vi "moveabs2.vi"(2 "SetPosition":sgl format="%.2f", 3 "EXP300 Axis":i8=1, 4 "THz Image\nESP Address":string="1:1") -> (0 "Current Position":dbl)   [LabVIEW 2010]
panel:
  out "Time to wait (s)":i16
  # "Stage Moving"
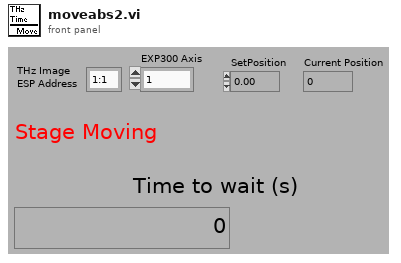
[diagram p1: front panel]
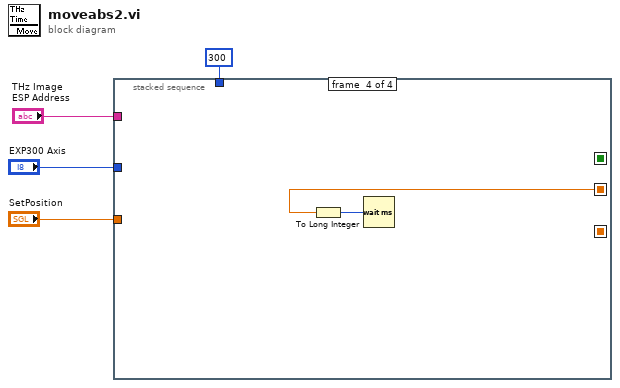
[diagram p0: block diagram]
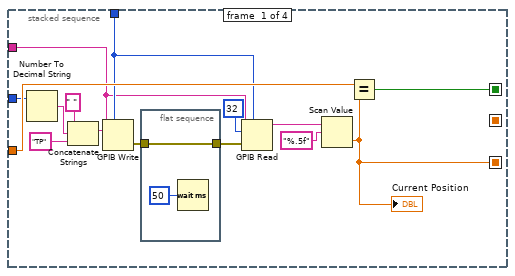
[diagram p2: hidden frame]
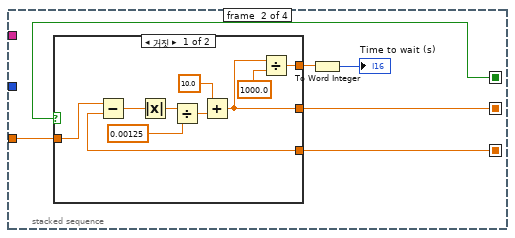
[diagram p3: hidden frame]
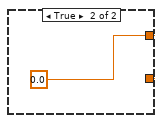
[diagram p4: hidden frame]
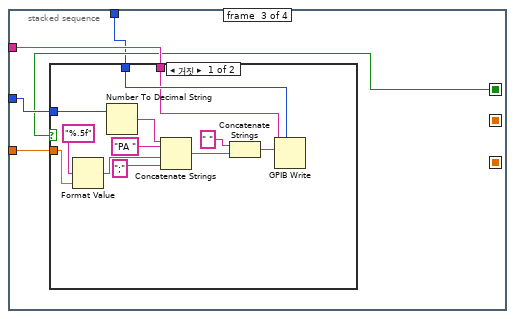
[diagram p5: hidden frame]
diagram:
  n1 = stacked-sequence {
    seq-local: [w18 _ _ _] -> [_ w26 _ _]
    seq-local: [w16 _ _ _] -> [_ w25 w40 _]
    seq-local: [_ w24 _ _] -> [_ _ _ w57]
    tunnel: "THz Image\nESP Address" -> [w5 _ w43 _]
    tunnel: "EXP300 Axis" -> [w13 _ w42 _]
    tunnel: "SetPosition" -> [w17 w27 w41 _]
    tunnel: 300 ("timeout ms (488.2 global)") -> [w11 _ w39 _]
    frame #0 {
      n2 = Number To Decimal String(number=w13) -> (decimal integer string=w7:string)  [unwired: 1 in]
      n3 = Concatenate Strings(" " ("string"), w7, "TP" ("string")) -> (w12:string)
      n4 = GPIB Write(0:w5, 1:w12, 4:w11) -> (6:w9:errorcluster)  [unwired: 2 in, 1 out]
      n5 = flat-sequence {
        tunnel: w9 -> [w21]
        tunnel: [w21] -> w8
        frame #0 {
          n6 = Wait (ms)(milliseconds to wait=u32 50) -> ()  [unwired: 1 out]
        }
      }
      n7 = GPIB Read(0:w5, 1:32 ("byte count"), 3:w8, 4:w11) -> (5:w15:string)  [unwired: 1 in, 2 out]
      n8 = Scan Value(string=w15, format string="%.5f") -> (value=w18:dbl)  [unwired: 1 in, 1 out]
      "Current Position" <- w18
      n9 = Equal?(x=w17, y=w18) -> (x = y?=w16:bool)
    }
    frame #1 {
      n10 = case shown="거짓" w25 {
        tunnel: w27 -> [w34 _]
        tunnel: w26 -> [w33 _]
        tunnel: [w29 w38] -> w23
        tunnel: [w28 w38] -> w24
        frame False {
          n11 = Subtract(x=w34, y=w33) -> (x-y=w35:dbl)
          n12 = Absolute Value(x=w35) -> (abs(x)=w36:dbl)
          n13 = Divide(x=w36, y=0.00125) -> (x/y=w32:dbl)
          n14 = Add(x=10.0, y=w32) -> (x+y=w28:dbl)
          n15 = Divide(x=w28, y=1000.0) -> (x/y=w29:dbl)
        }
        frame True {
          w38 = 0.0
        }
      }
      n16 = To Word Integer(number=w23) -> (16bit integer=→"Time to wait (s)":i16)
    }
    frame #2 {
      n17 = case shown="거짓" w40 {
        tunnel: w43 -> [w44 _]
        tunnel: w42 -> [w55 _]
        tunnel: w41 -> [w53 _]
        tunnel: w39 -> [w50 _]
        frame False {
          n18 = Format Value(format string="%.5f", value (0)=w53) -> (output string=w52:string)  [unwired: 1 in]
          n19 = Number To Decimal String(number=w55) -> (decimal integer string=w48:string)  [unwired: 1 in]
          n20 = Concatenate Strings(w48, "PA " ("string"), w52, ";" ("string")) -> (w47:string)
          n21 = Concatenate Strings(" " ("string"), w47) -> (w46:string)
          n22 = GPIB Write(0:w44, 1:w46, 4:w50) -> ()  [unwired: 2 in, 2 out]
        }
        frame True {
        }
      }
    }
    frame #3 {
      n23 = To Long Integer(number=w57) -> (32bit integer=w56:i32)
      n24 = Wait (ms)(milliseconds to wait=w56) -> ()  [unwired: 1 out]
    }
  }
